vi "Draw XY Data_modded.vi"(4 "[sized scatter plot cosmetics]":T2={"min size"=1, "max size"=5, "maps to max size"=5, "color array"=[16776960, 65280, 16711680, 255]}, 6 "xy cosmetics":T4={"plot color"=16776960, "plot type"=enum."connected points", "baseline"=0.0} {"baseline" format="%0.2f"}, 7 "pen":T1={"Width"=1, "Style"=enum."Solid"}, 8 "xy data":cluster{"x":dbl, "y":dbl}[](array[cluster]) {"y" format="%0.2f"; "x" format="%0.2f"}, 9 "y scale factors":cluster{"a":dbl, "b":dbl, "log?":bool} {"b" format="%0.2f"; "a" format="%0.2f"}, 10 "x scale factors":cluster{"a":dbl, "b":dbl, "log?":bool} {"b" format="%0.2f"; "a" format="%0.2f"}, 11 "picture":picture) -> (3 "new picture":picture)   [LabVIEW 2018]
uses:
  <vilib>/picture/cartesn2.llb/XY Plot Type.ctl
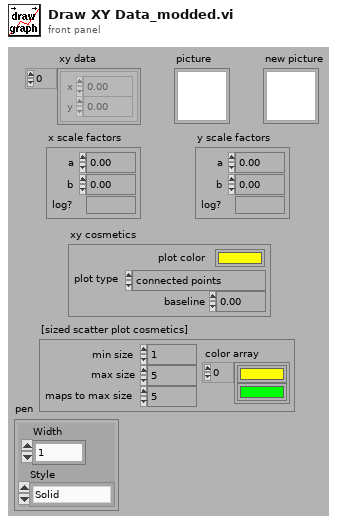
[diagram p1: front panel]
types:
  T1 = cluster{"Width":u16, "Style":enum32{"Solid", "Dash", "Dot", "DashDot", "DashDotDot"}}
  T2 = cluster{"min size":i16, "max size":i16, "maps to max size":i16, "color array":u32[]}
  T3 = typedef "XY Plot Type.ctl" = enum16{"points", "squares", "circles", "connected points", "connected squares", "connected circles", "comb plot", "sized scatter plot", "sized-colored scatter plot", "min-max lines"}
  T4 = cluster{"plot color":u32, "plot type":T3, "baseline":dbl}
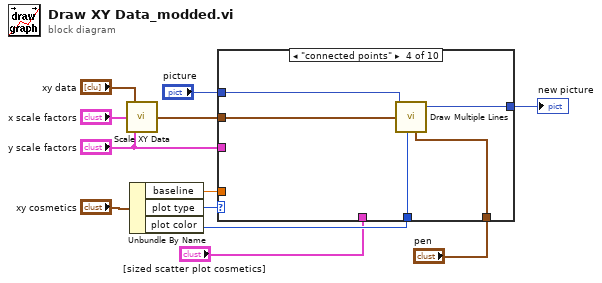
[diagram p0: block diagram]
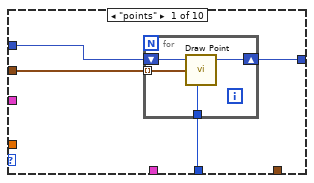
[diagram p2: hidden frame]
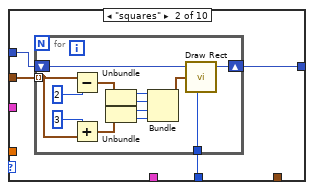
[diagram p3: hidden frame]
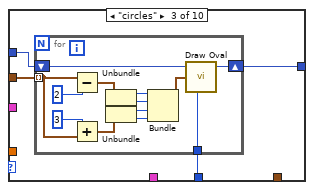
[diagram p4: hidden frame]
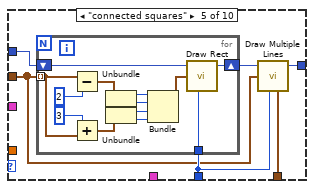
[diagram p5: hidden frame]
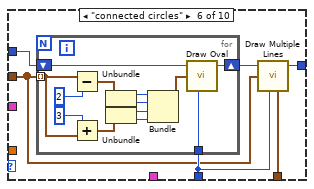
[diagram p6: hidden frame]
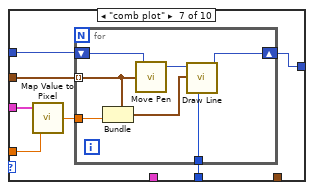
[diagram p7: hidden frame]
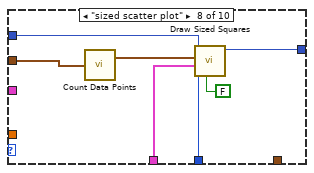
[diagram p8: hidden frame]
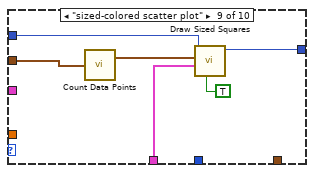
[diagram p9: hidden frame]
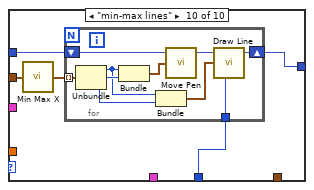
[diagram p10: hidden frame]
diagram:
  n1 = call <vilib>:"Scale XY Data.vi"("y scale factors"="y scale factors", "x scale factors"="x scale factors", "xy data"="xy data") -> ("scaled xy data"=w9:cluster{"x":i16, "y":i16}[])
  n2 = Unbundle By Name("xy cosmetics") -> ("baseline"=w4:dbl, "plot type"=w5:T3, "plot color"=w12:u32)
  n3 = case shown="\"connected points\"" w5 {
    tunnel: w12 -> [w16 w21 w38 w58 w65 w84 w98 w114 _ w128]
    tunnel: [w15 w22 w39 w59 w63 w82 w101 w118 w121 w125] -> w11
    tunnel: "picture" -> [w14 w23 w40 w56 w62 w81 w102 w115 w123 w129]
    tunnel: w9 -> [w13 w24 w41 w57 w61 w80 w100 w116 w124 w126]
    tunnel: w4 -> [_ _ _ _ _ _ w103 _ _ _]
    tunnel: "y scale factors" -> [_ _ _ _ _ _ w104 _ _ _]
    tunnel: "[sized scatter plot cosmetics]" -> [_ _ _ _ _ _ _ w113 w120 _]
    tunnel: "pen" -> [_ _ _ w55 w60 w79 _ _ _ _]
    frame "points" {
      n4 = for {
        shift-right: [w20] -> w15
        shift-left: w14 -> [w19]
        tunnel: w16 -> [w18]
        tunnel: w13 -> [w17] mode=indexing
        n5 = call <vilib>:"Draw Point.vi"("picture"=w19, "point(x,y)"=w17, "color(black)"=w18) -> ("new picture"=w20:picture)  [unwired: 6 in]
      }
    }
    frame "squares" {
      n6 = for {
        tunnel: w24 -> [w34] mode=indexing
        shift-right: [w37] -> w22
        shift-left: w23 -> [w36]
        tunnel: w21 -> [w35]
        n7 = Subtract(x=w34, y=i16 2) -> (x-y=w27:cluster{"x":i16, "y":i16})
        n8 = Add(x=i16 3, y=w34) -> (x+y=w33:cluster{"x":i16, "y":i16})
        n9 = Unbundle(w27) -> ("x"=w29:i16, "y"=w30:i16)
        n10 = Unbundle(w33) -> ("x"=w31:i16, "y"=w32:i16)
        n11 = Bundle("x"=w29, "y"=w30, "x"=w31, "y"=w32) -> (w28:cluster{"x":i16, "y":i16, "x":i16, "y":i16})  [unwired: 1 in]
        n12 = call <vilib>:"Draw Rect.vi"("picture"=w36, "rect"=w28, "color(black)"=w35) -> ("new picture"=w37:picture)  [unwired: 6 in]
      }
    }
    frame "circles" {
      n13 = for {
        tunnel: w41 -> [w51] mode=indexing
        shift-right: [w54] -> w39
        shift-left: w40 -> [w53]
        tunnel: w38 -> [w52]
        n14 = Subtract(x=w51, y=i16 2) -> (x-y=w44:cluster{"x":i16, "y":i16})
        n15 = Add(x=i16 3, y=w51) -> (x+y=w50:cluster{"x":i16, "y":i16})
        n16 = Unbundle(w44) -> ("x"=w46:i16, "y"=w47:i16)
        n17 = Unbundle(w50) -> ("x"=w48:i16, "y"=w49:i16)
        n18 = Bundle("x"=w46, "y"=w47, "x"=w48, "y"=w49) -> (w45:cluster{"x":i16, "y":i16, "x":i16, "y":i16})  [unwired: 1 in]
        n19 = call <vilib>:"Draw Oval.vi"("picture"=w53, "rect"=w45, "color(black)"=w52) -> ("new picture"=w54:picture)  [unwired: 6 in]
      }
    }
    frame "connected points" {
      n20 = call <vilib>:"Draw Multiple Lines.vi"("picture"=w56, "line endpoints"=w57, "color(black)"=w58, "pen"=w55) -> ("new picture"=w59:picture)  [unwired: 5 in]
    }
    frame "connected squares" {
      n21 = for {
        tunnel: w61 -> [w69] mode=indexing
        shift-right: [w78] -> w64
        shift-left: w62 -> [w77]
        tunnel: w65 -> [w71]
        n22 = Subtract(x=w69, y=i16 2) -> (x-y=w68:cluster{"x":i16, "y":i16})
        n23 = Add(x=i16 3, y=w69) -> (x+y=w70:cluster{"x":i16, "y":i16})
        n24 = Unbundle(w68) -> ("x"=w76:i16, "y"=w75:i16)
        n25 = Unbundle(w70) -> ("x"=w74:i16, "y"=w73:i16)
        n26 = Bundle("x"=w76, "y"=w75, "x"=w74, "y"=w73) -> (w72:cluster{"x":i16, "y":i16, "x":i16, "y":i16})  [unwired: 1 in]
        n27 = call <vilib>:"Draw Rect.vi"("picture"=w77, "rect"=w72, "color(black)"=w71) -> ("new picture"=w78:picture)  [unwired: 6 in]
      }
      n28 = call <vilib>:"Draw Multiple Lines.vi"("picture"=w64, "line endpoints"=w61, "color(black)"=w65, "pen"=w60) -> ("new picture"=w63:picture)  [unwired: 5 in]
    }
    frame "connected circles" {
      n29 = for {
        tunnel: w80 -> [w88] mode=indexing
        shift-right: [w97] -> w83
        shift-left: w81 -> [w96]
        tunnel: w84 -> [w90]
        n30 = Subtract(x=w88, y=i16 2) -> (x-y=w87:cluster{"x":i16, "y":i16})
        n31 = Add(x=i16 3, y=w88) -> (x+y=w89:cluster{"x":i16, "y":i16})
        n32 = Unbundle(w87) -> ("x"=w95:i16, "y"=w94:i16)
        n33 = Unbundle(w89) -> ("x"=w93:i16, "y"=w92:i16)
        n34 = Bundle("x"=w95, "y"=w94, "x"=w93, "y"=w92) -> (w91:cluster{"x":i16, "y":i16, "x":i16, "y":i16})  [unwired: 1 in]
        n35 = call <vilib>:"Draw Oval.vi"("picture"=w96, "rect"=w91, "color(black)"=w90) -> ("new picture"=w97:picture)  [unwired: 6 in]
      }
      n36 = call <vilib>:"Draw Multiple Lines.vi"("picture"=w83, "line endpoints"=w80, "color(black)"=w84, "pen"=w79) -> ("new picture"=w82:picture)  [unwired: 5 in]
    }
    frame "comb plot" {
      n37 = call <vilib>:"Map Value to Pixel.vi"("x"=w103, "scale factors"=w104) -> ("pixel"=w99:dbl)  [unwired: 1 in]
      n38 = for {
        shift-right: [w109] -> w101
        shift-left: w102 -> [w111]
        tunnel: w100 -> [w107] mode=indexing
        tunnel: w99 -> [w108]
        tunnel: w98 -> [w105]
        n39 = Bundle(cluster=w107, "y"=w108) -> (w106:cluster{"x":i16, "y":i16})  [unwired: 1 in]
        n40 = call <vilib>:"Move Pen.vi"("new position"=w107, "picture"=w111) -> ("new picture"=w110:picture)  [unwired: 3 in]
        n41 = call <vilib>:"Draw Line.vi"("picture"=w110, "end point"=w106, "color(black)"=w105) -> ("new picture"=w109:picture)  [unwired: 6 in]
      }
    }
    frame "sized scatter plot" {
      n42 = call <vilib>:"Count Data Points.vi"("scaled xy data"=w116) -> ("counted data"=w117:cluster{"x":i16, "y":i16, "c":i16}[])  [unwired: 1 out]
      n43 = call <vilib>:"Draw Sized Squares.vi"("multi-color(F)"=FALSE, "color(yellow)"=w114, "sized scatter plot cosmetics"=w113, "data"=w117, "picture"=w115) -> ("new picture"=w118:picture)  [unwired: 6 in]
    }
    frame "sized-colored scatter plot" {
      n44 = call <vilib>:"Count Data Points.vi"("scaled xy data"=w124) -> ("counted data"=w122:cluster{"x":i16, "y":i16, "c":i16}[])  [unwired: 1 out]
      n45 = call <vilib>:"Draw Sized Squares.vi"("multi-color(F)"=TRUE, "sized scatter plot cosmetics"=w120, "data"=w122, "picture"=w123) -> ("new picture"=w121:picture)  [unwired: 7 in]
    }
    frame "min-max lines" {
      n46 = call <vilib>:"Min Max X.vi"("scaled xy data"=w126) -> ("min max data"=w127:cluster{"x":i16, "min":i16, "max":i16}[])
      n47 = for {
        shift-right: [w139] -> w125
        shift-left: w129 -> [w136]
        tunnel: w127 -> [w135] mode=indexing
        tunnel: w128 -> [w138]
        n48 = Unbundle(w135) -> ("x"=w131:i16, "min"=w133:i16, "max"=w132:i16)
        n49 = Bundle("x"=w131, "min"=w133) -> (w130:cluster{"x":i16, "min":i16})  [unwired: 1 in]
        n50 = Bundle("x"=w131, "max"=w132) -> (w134:cluster{"x":i16, "max":i16})  [unwired: 1 in]
        n51 = call <vilib>:"Move Pen.vi"("new position"=w130, "picture"=w136) -> ("new picture"=w137:picture)  [unwired: 3 in]
        n52 = call <vilib>:"Draw Line.vi"("picture"=w137, "end point"=w134, "color(black)"=w138) -> ("new picture"=w139:picture)  [unwired: 6 in]
      }
    }
  }
  "new picture" <- w11
